vi "XIPIN_IBERT_7_Series_GTZ_3_1.vi"   [LabVIEW 2017]
doc: "The IBERT 7 Series GTZ core is customizable and designed for evaluating and monitoring 7 Series FPGA GTZ transceivers. This core includes pattern generators and checkers that are implemented in FPGA logic, and access to ports and the dynamic reconfiguration port attributes of the GTZ transceivers. Communication logic is also included to allow the design to be run-time accessible through Joint Test Action Group (JTAG). Run-time interaction with this core requires the use of the Vivado serial I/O analyzer feature.\n------------------------------------\n<b>Need License</b> : No"
uses:
  <vilib>/rvi/XilinxIP/XIPIN_XNode/niFpgaXIPIN.xnode
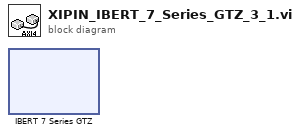
[diagram p0: block diagram]
diagram:
  n1 = xnode ("IBERT 7 Series GTZ")() -> ()
